vi "Created Queues.vi"(8 "Created Queue Alias":string, 9 "Priority?":bool, 10 "Msg Strategy":refnum<class "Msg Strategy.lvclass">, 11 "Template Queue in":refnum<class "Template Queue.lvclass">) -> (3 "Template Queue out":refnum<class "Template Queue.lvclass">)   [LabVIEW 2021, in "_Template.lvlib" / "Templates.lvlib" / "Template Queue.lvlib" / "Template Queue.lvclass"]
uses:
  <vilib>/jettl/jettl/jettl/Msg Strategy/Msg Strategy.lvclass
  Template Queue.lvclass
  Template Queue.lvclass/Template Queue.ctl
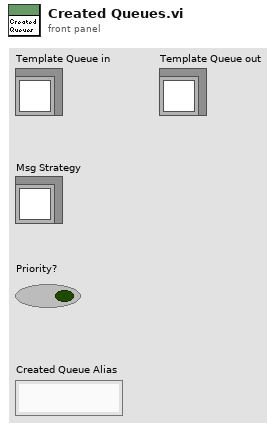
[diagram p1: front panel]
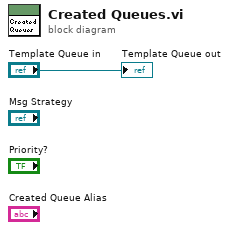
[diagram p0: block diagram]
diagram:
  "Template Queue out" <- "Template Queue in"
